vi "Battery Statuses to Dashboard.vi"(1 "Battery Status":T2, 2 "BMS Low Voltage Status":T3 {"Temp. 0" scale=0.0..80.0; "Temp. 1" scale=0.0..80.0}, 3 "Dashboard Control in":T1={"Tractive System"=TRUE, "RTD"=TRUE, "AMS error"=TRUE, "IMD error"=TRUE, "Low Voltage"=0.0, "High Voltage"=0.0} {"High Voltage" scale=0.0..10.0; "Low Voltage" scale=0.0..10.0}) -> (0 "Dashboard Control out":T1={"Tractive System"=TRUE, "RTD"=TRUE, "AMS error"=TRUE, "IMD error"=TRUE, "Low Voltage"=0.0, "High Voltage"=0.0} {"High Voltage" scale=0.0..10.0; "Low Voltage" scale=0.0..10.0})   [LabVIEW 2016]
uses:
  Users/s163601/Desktop/05-28/RT/BMS Voltage status 2.ctl
  Users/s163601/Desktop/05-28/RT/Battery Status.ctl
  Users/s163601/Desktop/05-28/Tests/Dashboard Control.ctl
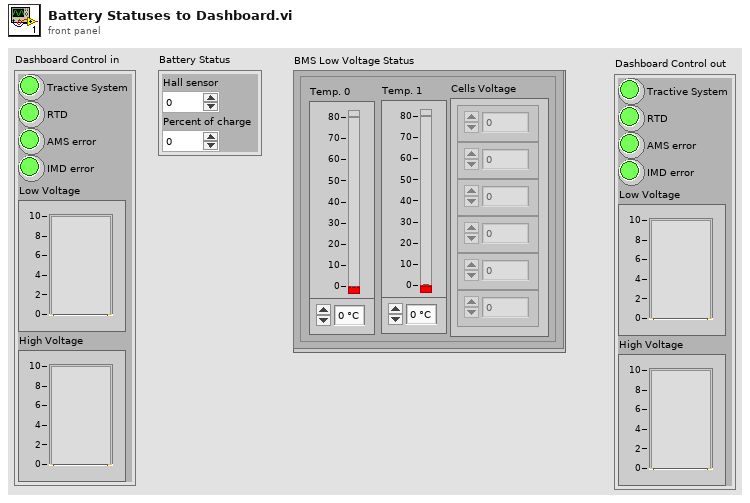
[diagram p1: front panel]
types:
  T1 = typedef "Dashboard Control.ctl" = cluster{"Tractive System":bool, "RTD":bool, "AMS error":bool, "IMD error":bool, "Low Voltage":dbl, "High Voltage":dbl}
  T2 = typedef "Battery Status.ctl" = cluster{"Hall sensor":i32, "Percent of charge":i16}
  T3 = typedef "BMS Voltage status 2.ctl" = cluster{"Cells Voltage":dbl[], "Temp. 1":u8, "Temp. 0":u8}
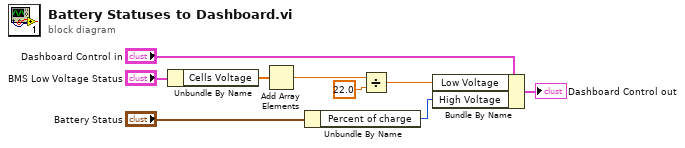
[diagram p0: block diagram]
diagram:
  n1 = Unbundle By Name("BMS Low Voltage Status") -> ("Cells Voltage"=w2:dbl[])
  n2 = Add Array Elements(numeric array=w2) -> (sum=w1:dbl)
  n3 = Unbundle By Name("Battery Status") -> ("Percent of charge"=w3:i16)
  n4 = Divide(x=w1, y=22.0) -> (x/y=w8:dbl)
  n5 = Bundle By Name(cluster="Dashboard Control in", "Low Voltage"=w8, "High Voltage"=w3) -> (→"Dashboard Control out":T1)
